vi "GenerateInterleavedList.vi"(4 "# passes":i32, 5 "# points":i32, 6 "Stop":dbl, 7 "Start":dbl) -> (2 "Array":dbl[](array[numeric]), 3 "Points per pass":i32)   [LabVIEW 2018]
uses:
  <vilib>/Analysis/1siggen.llb/Ramp Pattern by Samples.vi
  <vilib>/Analysis/NI_AALBase.lvlib
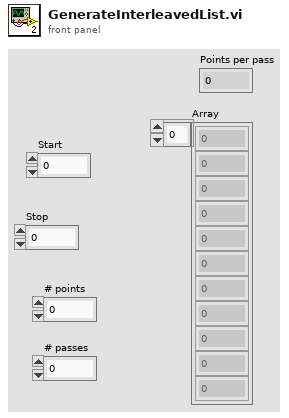
[diagram p1: front panel]
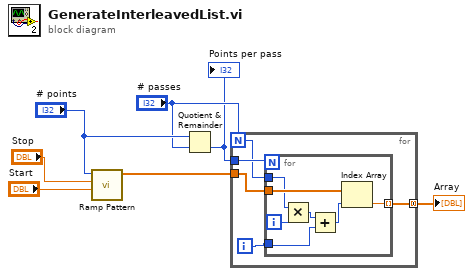
[diagram p0: block diagram]
diagram:
  n1 = call-poly <vilib>:"Ramp Pattern.vi"("start"="Start", "end"="Stop", "samples"="# points") -> ("Ramp Pattern"=w3:dbl[])  [unwired: 7 in, 1 out]
  n2 = Quotient & Remainder(x="# points", y="# passes") -> (floor(x/y)=w2:i32)  [unwired: 1 out]
  "Points per pass" <- w2
  n3 = for {
    N: "# passes" -> [w9]
    tunnel: w3 -> [w11]
    tunnel: w2 -> [w12]
    tunnel: [w10] -> w1 mode=concatenating
    i -> [w8]
    n4 = for {
      N: w12 -> [_]
      tunnel: w11 -> [w19]
      tunnel: [w18] -> w10 mode=indexing
      tunnel: w9 -> [w17]
      tunnel: w8 -> [w14]
      i -> [w16]
      n5 = Multiply(x=w17, y=w16) -> (x*y=w15:i32)
      n6 = Add(x=w15, y=w14) -> (x+y=w13:i32)
      n7 = Index Array(array=w19, index=w13) -> (element=w18:dbl)
    }
  }
  "Array" <- w1
